vi "Construct Sequence.vi"(8 "error in":errorcluster, 11 "P Cal Builder in":refnum<class "P Cal Builder.lvclass">) -> (0 "error out":errorcluster, 2 "New Sequence":refnum<class "SEQ.lvclass">, 3 "P Cal Builder out":refnum<class "P Cal Builder.lvclass">)   [LabVIEW 2015, in "P Cal Builder.lvclass"]
doc: "Construct a new sequence using the builder class."
uses:
  P Cal Builder.lvclass
  Reusable/Sequence/SEQ/SEQ.lvclass
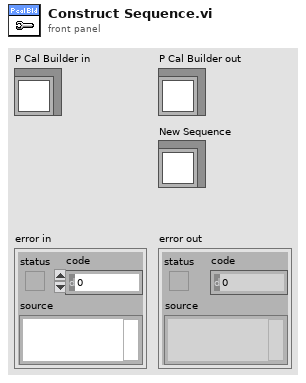
[diagram p1: front panel]
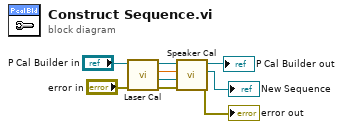
[diagram p0: block diagram]
diagram:
  n1 = call "Laser Cal.vi"("error in"="error in", "P Cal Builder in"="P Cal Builder in") -> ("error out"=w4:errorcluster, "SEQ out"=w5:refnum<class "SEQ.lvclass">, "Pfinal"=w8:dbl, "P Cal Builder out"=w6:refnum<class "P Cal Builder.lvclass">)  [unwired: 6 in]
  n2 = call "Speaker Cal.vi"("error in"=w4, "SEQ in"=w5, "Plow"=w8, "P Cal Builder in"=w6) -> ("error out"=→"error out":errorcluster, "SEQ out"=→"New Sequence":refnum<class "SEQ.lvclass">, "P Cal Builder out"=→"P Cal Builder out":refnum<class "P Cal Builder.lvclass">)  [unwired: 5 in]
